vi "Printer Dialog.vi"(8 "error in (no error)":errorcluster, 10 "VI Reference":refnum<vi>) -> (0 "error out":errorcluster, 1 "Cancelled":bool)   [LabVIEW 2020]
uses:
  System.Windows.Forms
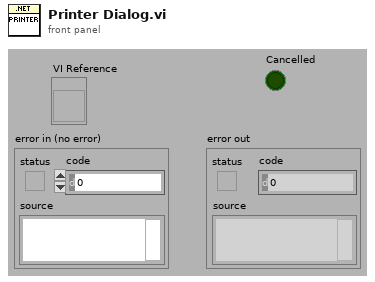
[diagram p1: front panel]
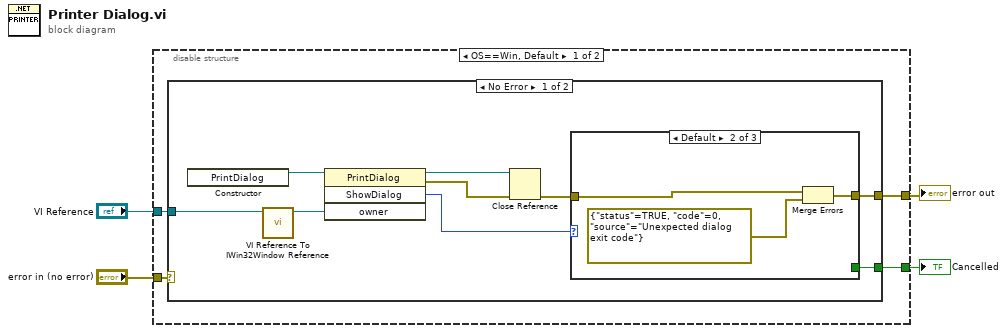
[diagram p0: block diagram]
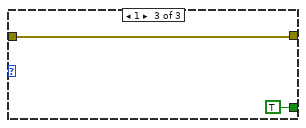
[diagram p3: hidden frame]
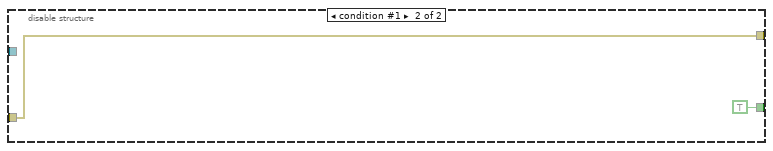
[diagram p5: hidden frame]
diagram:
  n1 = disable-structure shown="OS==Win, Default" {
    disable-tunnel: [w8 w26] -> w4
    disable-tunnel: "error in (no error)" -> [w7 w26]
    disable-tunnel: [w6 TRUE] -> w2
    disable-tunnel: "VI Reference" -> [w5 _]
    frame condition #0 (active) {
      n2 = case shown="No Error" w7 {
        selector: w7 -> [_ w25]
        tunnel: [w15 w25] -> w8
        tunnel: [w14 _] -> w6
        tunnel: w5 -> [w10 _]
        frame No Error {
          n3 = constructor class="PrintDialog"() -> (reference out=w17:refnum<k24>)  [unwired: 3 in, 2 out]
          n4 = call "VI Reference To IWin32Window Reference.vi"("VI Reference"=w10) -> ("System.Windows.Forms.IWin32Window"=w9:refnum<k24>)  [unwired: 9 in, 1 out]
          n5 = invoke class="PrintDialog" method="ShowDialog"(reference=w17, "owner"=w9) -> (reference out=w13:refnum<k24>, error out=w12:errorcluster, "ShowDialog"=w16:i32)  [unwired: 2 in, 1 out]
          n6 = Close Reference(reference=w13, error in (no error)=w12) -> (error out=w11:errorcluster)
          n7 = case shown="Default" w16 {
            tunnel: w11 -> [w18 w22 w23]
            tunnel: [w18 w20 w23] -> w15
            tunnel: [TRUE _ TRUE] -> w14
            frame 2 {
              # "Cancelled"
            }
            frame Default {
              n8 = Merge Errors(w22, errorcluster {"status"=TRUE, "code"=0, "source"="Unexpected dialog exit code"} ("error in 2 (no error)")) -> (w20:errorcluster)
            }
            frame 1 {
            }
          }
        }
        frame Error {
        }
      }
    }
    frame condition #1 {
    }
  }
  "error out" <- w4
  "Cancelled" <- w2
